vi "Search DB for Chars or Meas.vi"(6 "Windows? (F)":bool, 7 "Item Type":T1=enum."Measurement", 8 "error in (no error)":errorcluster, 10 "DB Path":path, 11 "Custom Device Node in":refnum<k24>) -> (0 "error out":errorcluster, 2 "Chans":string[](array[string]), 3 "Custom Device Node out":refnum<k24>)   [LabVIEW 2011]
uses:
  NationalInstruments.VeriStand.SystemStorage
  <vilib>/ECUMC/NIVS/Support Files.llb/Item Type.ctl
  <vilib>/ECUMC/ECUMC.llb/MC Get Names Type.ctt
  <vilib>/ECUMC/ECUMC.llb/MC Get Prop Char Dimension.vi
  <vilib>/ECUMC/ECUMC.lvlib
  <vilib>/ECUMC/NIVS/Support Files.llb/XCP and CCP Master Custom Device.lvlib
panel:
  in  "ECU name":string
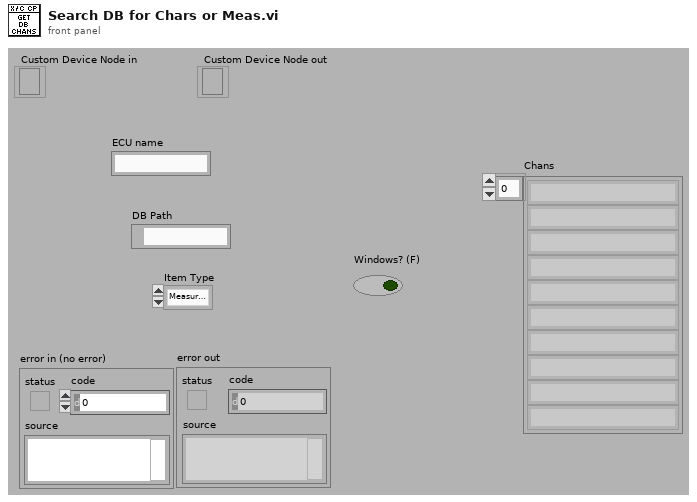
[diagram p1: front panel]
types:
  T1 = typedef "XCP and CCP Master Custom Device.lvlib/Item Type.ctl" = enum16{"Scalar Characteristic", "Curve Characteristic", "Field Characteristic", "Measurement"}
  T2 = typedef "ECUMC.lvlib/MC Get Names Type.ctt" = u32
  T3 = typedef "ECUMC.lvlib/MC Reference.ctt" = u32
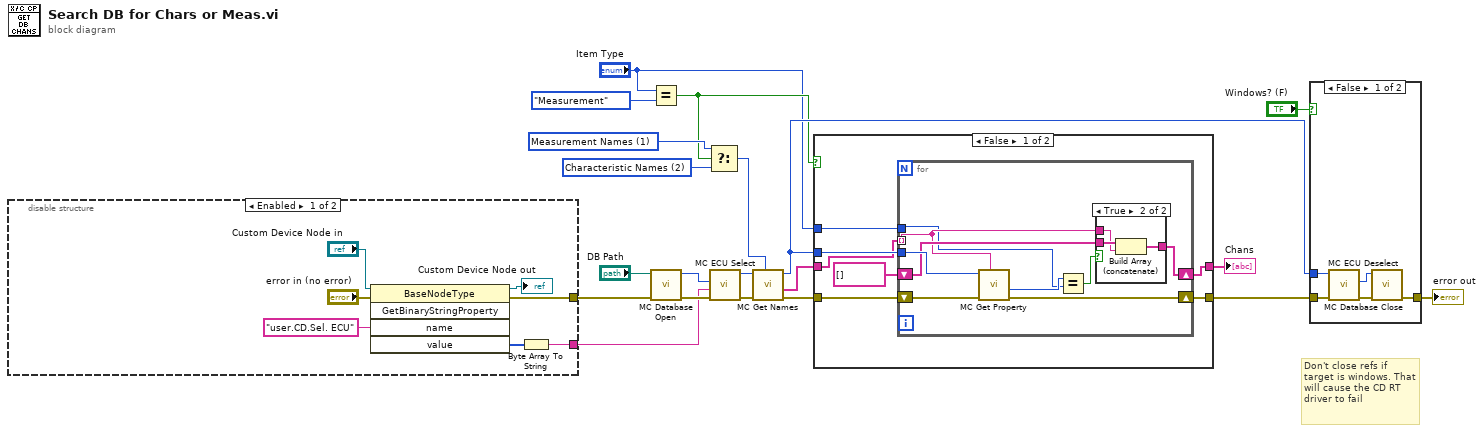
[diagram p0: block diagram]
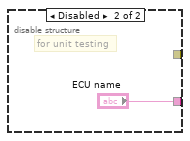
[diagram p2: hidden frame]
diagram:
  w19 = T2 1 items=["ECU Names", "Measurement Names", "Characteristic Names", "Event Channel Names", "Defined Pages Names"] ("type")
  w18 = T2 2 items=["ECU Names", "Measurement Names", "Characteristic Names", "Event Channel Names", "Defined Pages Names"] ("type")
  # "Don't close refs if target is windows. That will cause the CD RT driver to fail"
  n1 = disable-structure shown="Enabled" {
    disable-tunnel: [w25 _] -> w14
    disable-tunnel: [w21 "ECU name"] -> w11
    frame Enabled {
      n2 = invoke class="BaseNodeType" method="GetBinaryStringProperty"(reference="Custom Device Node in", error in="error in (no error)", "name"="user.CD.Sel. ECU") -> (reference out=→"Custom Device Node out":refnum<k24>, error out=w25:errorcluster, "value"=w23:u8[])  [unwired: 2 in, 2 out]
      n3 = Byte Array To String(unsigned byte array=w23) -> (string=w21:string)
    }
    frame Disabled {
      # "for unit testing"
    }
  }
  n4 = Equal?(x="Item Type", y=Item_Type."Measurement") -> (x = y?=w2:bool)
  n5 = call <vilib>:"MC Database Open.vi"("error in"=w14, "DB path"="DB Path") -> ("error out"=w13:errorcluster, "DB ref out"=w12:T3)  [unwired: 8 in]
  n6 = Select(t=w19, s=w2, f=w18) -> (s? t:f=w20:T2)
  n7 = call <vilib>:"MC ECU Select.vi"("error in"=w13, "ECU name"=w11, "DB ref in"=w12) -> ("error out"=w16:errorcluster, "ECU ref out"=w17:T3)  [unwired: 7 in]
  n8 = call <vilib>:"MC Get Names.vi"("type"=w20, "error in"=w16, "reference in"=w17) -> ("error out"=w10:errorcluster, "names list out"=w9:string[], "reference out"=w5:T3)  [unwired: 6 in]
  n9 = case shown="False" w2 {
    tunnel: w10 -> [w34 w49]
    tunnel: w5 -> [w33 _]
    tunnel: w9 -> [w32 w50]
    tunnel: [w31 w50] -> w8
    tunnel: [w30 w49] -> w7
    tunnel: "Item Type" -> [w29 _]
    frame False {
      n10 = for {
        tunnel: w32 -> [w39] mode=indexing
        tunnel: w33 -> [w44]
        shift-right: [w42] -> w30
        shift-left: w34 -> [w43]
        shift-right: [w38] -> w31
        shift-left: string[] [] -> [w40]
        tunnel: w29 -> [w36]
        n11 = call-poly <vilib>:"MC Get Property.vi"("name"=w39, "error in"=w43, "reference in"=w44) -> ("error out"=w42:errorcluster, "char dimension"=w41:u32)  [unwired: 6 in, 1 out]
        n12 = Equal?(x=w41, y=w36) -> (x = y?=w37:bool)
        n13 = case shown="True" w37 {
          tunnel: w40 -> [w45 w48]
          tunnel: w39 -> [_ w47]
          tunnel: [w45 w46] -> w38
          frame False {
          }
          frame True {
            n14 = Build Array (concatenate)(w48, w47) -> (w46:string[])
          }
        }
      }
    }
    frame True {
    }
  }
  "Chans" <- w8
  n15 = case shown="False" "Windows? (F)" {
    tunnel: w7 -> [w55 w56]
    tunnel: w5 -> [w53 _]
    tunnel: [w51 w56] -> w4
    frame False {
      n16 = call <vilib>:"MC ECU Deselect.vi"("error in"=w55, "ECU ref in"=w53) -> ("error out"=w54:errorcluster, "DB ref out"=w52:T3)  [unwired: 8 in]
      n17 = call <vilib>:"MC Database Close.vi"("error in"=w54, "DB ref in"=w52) -> ("error out"=w51:errorcluster)  [unwired: 9 in]
    }
    frame True {
    }
  }
  "error out" <- w4
